vi "example_10_error.vi"() -> ()   [LabVIEW 2015, in "lv-dialog.lvlib" / "v1.lvlib"]
uses:
  v1.lvlib
  public/_controls/dialog_selection.ctl
  <vilib>/Utility/error.llb/Error Cluster From Error Code.vi
  <vilib>/ErrorRing/Error Ring.xnode
  public/class/v1.lvclass
panel:
  in  "error in":errorcluster
  out "error out":errorcluster
  out "dialog_selection":T1
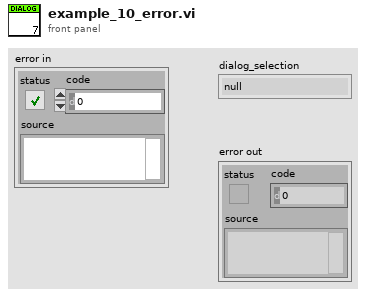
[diagram p1: front panel]
types:
  T1 = typedef "lv-dialog.lvlib/v1.lvlib/dialog_selection.ctl" = enum16{"null", "panel_closed", "button_1", "button_2", "button_3", "cancelled"}
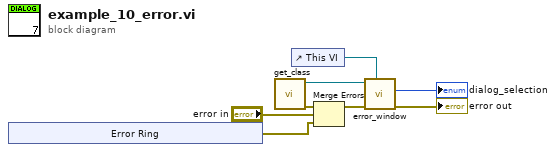
[diagram p0: block diagram]
diagram:
  n1 = xnode "Error Ring"() -> ("error out"=w1:errorcluster)
  n2 = call "get_class.vi"() -> ("error out"=w5:errorcluster, "class"=w4:refnum<class "v1.lvclass">)  [unwired: 10 in]
  n3 = control-ref of="This VI"() -> (w8:refnum<vi>)
  n4 = Merge Errors(w5, "error in", w1) -> (w3:errorcluster)
  n5 = call-dynamic "error_window.vi"("callee"=w8, "error in (no error)"=w3, "v1 in"=w4) -> ("error out"=→"error out":errorcluster, "dialog_selection"=→"dialog_selection":T1)  [unwired: 6 in, 1 out]
